vi "Learning about Qs.vi"() -> ()   [LabVIEW 2021]
panel:
  out "Iteration":i32
  out "Numeric Indicator":i32
  in  "Numeric Control":i32
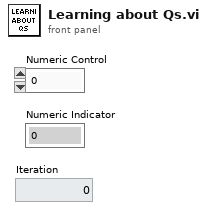
[diagram p1: front panel]
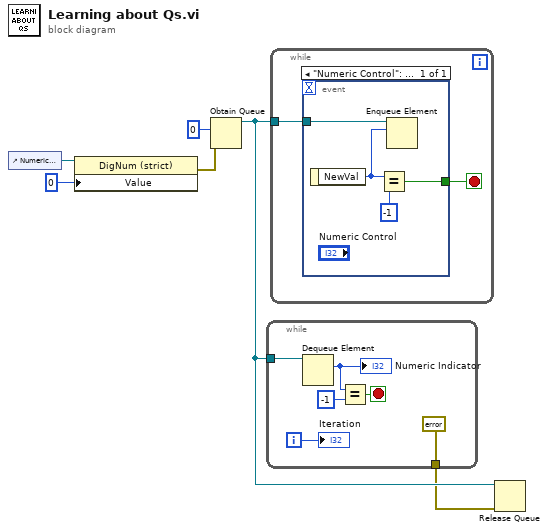
[diagram p0: block diagram]
diagram:
  n1 = control-ref of="Numeric Control"() -> (w6:refnum<vi>)
  n2 = property class="DigNum (strict)"(reference=w6, "Value"=0) -> (error out=w5:errorcluster)  [unwired: 1 in, 1 out]
  n3 = Obtain Queue(element data type=0 ("Value"), error in (no error)=w5) -> (queue out=w3:refnum<queue>)  [unwired: 3 in, 2 out]
  n4 = while {
    tunnel: w3 -> [w7]
    tunnel: [errorcluster {"status"=FALSE, "code"=0, "source"=""} ("error in (no error)")] -> w2
    i -> [w12]
    stop <- w11 stop-if-true
    n5 = Dequeue Element(queue=w7) -> (element=w9:i32)  [unwired: 2 in, 3 out]
    "Numeric Indicator" <- w9
    n6 = Equal?(x=w9, y=-1) -> (x = y?=w11:bool)
    "Iteration" <- w12
  }
  n7 = while {
    tunnel: w3 -> [w13]
    stop <- w14 stop-if-true
    n8 = event shown="[0] \"Numeric Control\": Value Change" {
      selector: _ -> [_]
      dyn-events: _ -> [_]
      timeout: _ -> [_]
      tunnel: w13 -> [w15]
      tunnel: [w17] -> w14
      event "Numeric Control": Value Change {
        n9 = event-data() -> ("NewVal"=w16:i32)  [unwired: 1 in]
        n10 = Equal?(x=w16, y=-1) -> (x = y?=w17:bool)
        n11 = Enqueue Element(queue=w15, element=w16) -> ()  [unwired: 2 in, 3 out]
      }
    }
  }
  n12 = Release Queue(queue=w3, error in (no error)=w2) -> ()  [unwired: 1 in, 3 out]
